vi "Robot Main.vi"() -> ()   [LabVIEW 2016]
doc: "This VI implements the framework and scheduler for your robotics program. It should not be necessary to modify the framework. You are expected to add your code to the VIs called from Robot Main - the ones located in the Team Code folder within the project."
uses:
  <vilib>/Rock Robotics/WPI/Camera/WPI_CameraImageSize.ctl
  NavX/_TypeDefs/FRIC_navX_DeviceNumbersTypeDef.ctl
  NavX/_TypeDefs/Z900_navX_SerialStreamTypeDef.ctl
  NavX/_Processing Loop/FRIC_navX_Internal_SPI_ProcessingLoop.vi
  NavX/_Processing Loop/FRIC_navX_Internal_USB_ProcessingLoop.vi
  _Support Files/Robot Global Data.vi
panel:
  in  "Image Size":T1=enum."320x240"
  in  "Enable Vision":bool
  in  "Finish":bool
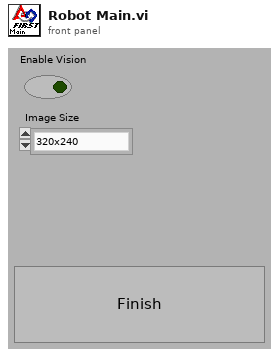
[diagram p1: front panel]
types:
  T1 = typedef "WPI_CameraImageSize.ctl" = enum16{"640x480", "320x240", "160x120", "Custom"}
  T2 = typedef "Z900_navX_SerialStreamTypeDef.ctl" = enum16{"YRPH", "Quaterinons", "Gyro/Raw", "AHRS", "AHRSAndPositioning"}
  T3 = typedef "FRIC_navX_DeviceNumbersTypeDef.ctl" = enum16{"Dev0", "Dev1", "Dev2", "Dev3", "Dev4", "Dev5", "Dev6", "Dev7", "Dev8", "Dev9", "Dev10"}
  T4 = typedef "WPI_DriverStationMatch Info.ctl" = cluster{"Autonomous Elapsed Seconds":dbl, "TeleOp Elapsed Seconds":dbl, "Disabled Elapsed Seconds":dbl, "Visited Autonomous":bool, "Visited TeleOp":bool, "Visited Disabled":bool, "Autonomous Settings":cluster{"Autonomous Style":enum16{"Iterative", "Independent"}, "VI Refnum":refnum<vi>}}
  T5 = typedef "WPI_DriverStationDerivedRobotMode.ctl" = enum16{"Init", "Execute", "Stop"}
  T6 = typedef "WPI_DriverStationRobotMode2.ctl" = enum16{"Autonomous Disabled", "Autonomous Enabled", "Teleop Disabled", "Teleop Enabled", "Disconnected", "Finish", "Test Disabled", "Test Enabled", "Emergency Stopped"}
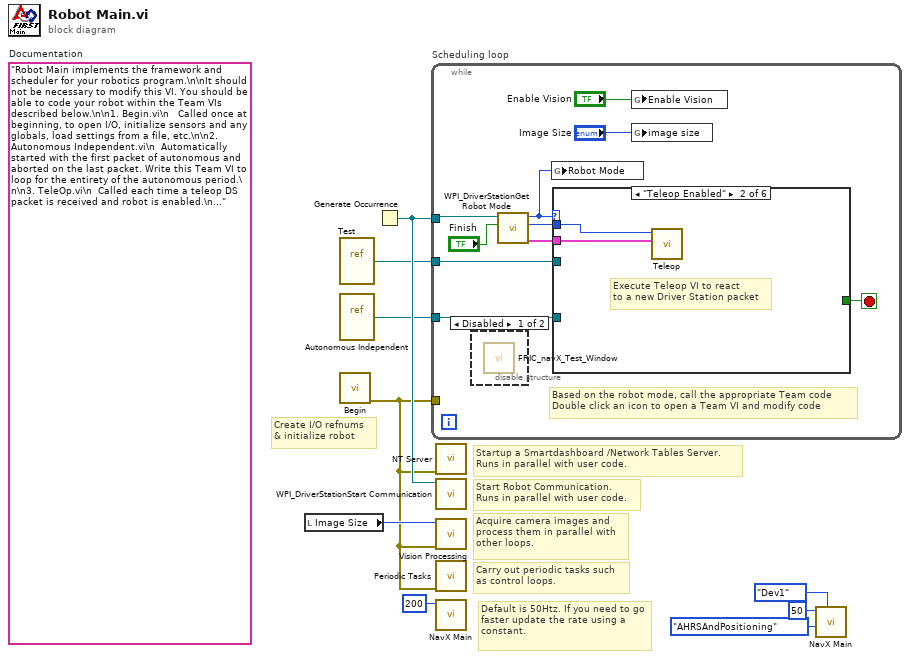
[diagram p0: block diagram]
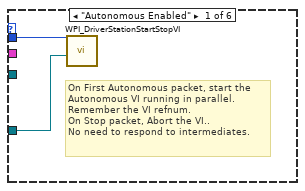
[diagram p3: hidden frame]
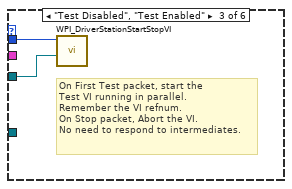
[diagram p4: hidden frame]
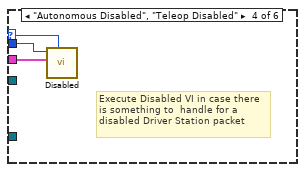
[diagram p5: hidden frame]
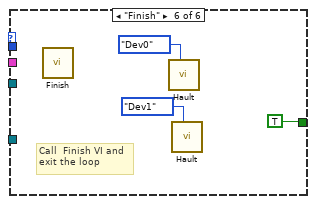
[diagram p7: hidden frame]
diagram:
  (unwired) "Robot Main implements the framework and scheduler for your robotics program.\n\nIt should not be necessary to modify this VI. You should be able to code your robot within the Team VIs described below.\n\n1. Begin.vi\n   Called once at beginning, to open I/O, initialize sensors and any globals, load settings from a file, etc.\n\n2. Autonomous Independent.vi\n  Automatically started with the first packet of autonomous and aborted on the last packet. Write this Team VI to loop for the entirety of the autonomous period.\n\n3. TeleOp.vi\n  Called each time a teleop DS packet is received and robot is enabled.\n\n4. Disabled.vi\n  Called each time a packet is received and the robot is disabled.\n\n5. Test.vi\n  Called Automatically started with the first test packet and aborted on the last. Modify this VI to carry out robot and sensor validation tests.\n\n6. Vision.vi\n  A parallel loop that acquires and processes camera images.\n\n7. PeriodicTasks.vi\n  Parallel loops running at user-defined rates.\n\n8. Finish.vi\n  Called before exiting, so you can save data, clean up I/O, etc.\n"  # Documentation
  # "Default is 50Htz. If you need to go faster update the rate using a constant."
  # "Startup a Smartdashboard /Network Tables Server.\nRuns in parallel with user code."
  # "Carry out periodic tasks such\nas control loops."
  # "Acquire camera images and\nprocess them in parallel with\nother loops."
  # "Create I/O refnums\n& initialize robot"
  # "Start Robot Communication.\nRuns in parallel with user code."
  n1 = local read "Image Size"() -> (w6:T1)
  n2 = vi-ref "Test.vi"() -> (w7:refnum<vi>)
  n3 = vi-ref "Autonomous Independent.vi"() -> (w8:refnum<vi>)
  n4 = call "Begin.vi"() -> ("error out"=w4:errorcluster)  [unwired: 1 in, 10 out]
  n5 = Generate Occurrence() -> (w9:refnum<k4>)
  n6 = while "Scheduling loop" {
    tunnel: w9 -> [w18]
    tunnel: w4 -> [_]
    tunnel: w8 -> [w13]
    tunnel: w7 -> [w11]
    stop <- w15 stop-if-true
    # "Based on the robot mode, call the appropriate Team code\nDouble click an icon to open a Team VI and modify code"
    n7 = disable-structure shown="Disabled" {
      frame Disabled {
        n8 = call "FRIC_navX_Test_Window.vi"() -> ()  [unwired: 12 in]
      }
      frame Enabled {
      }
    }
    n9 = call <vilib>:"WPI_DriverStationGet Robot Mode.vi"("Finish"="Finish", "DS Occurrence"=w18) -> ("Match Info out"=w16:T4, "Call Context"=w19:T5, "Robot Mode"=w10:T6)  [unwired: 7 out]
    n10 = global write "Robot Global Data.vi" "Robot Mode"(w10) -> ()
    n11 = case shown="\"Teleop Enabled\"" w10 {
      selector: w10 -> [_ _ _ w26 _ _]
      tunnel: w19 -> [w21 w23 w25 w28 _ _]
      tunnel: w16 -> [_ w22 _ w27 _ _]
      tunnel: [_ _ _ _ _ TRUE] -> w15
      tunnel: w13 -> [w20 _ _ _ _ _]
      tunnel: w11 -> [_ _ w24 _ _ _]
      frame "Autonomous Enabled" {
        # "On First Autonomous packet, start the\nAutonomous VI running in parallel.\nRemember the VI refnum.\nOn Stop packet, Abort the VI..\nNo need to respond to intermediates."
        n12 = call <vilib>:"WPI_DriverStationStartStopVI.vi"("VI in"=w20, "Call Context"=w21) -> ()  [unwired: 10 in]
      }
      frame "Teleop Enabled" {
        # "Execute Teleop VI to react\nto a new Driver Station packet"
        n13 = call "Teleop.vi"("Match Info"=w22, "Call Context"=w23) -> ()  [unwired: 1 in, 9 out]
      }
      frame "Test Disabled", "Test Enabled" {
        # "On First Test packet, start the\nTest VI running in parallel.\nRemember the VI refnum.\nOn Stop packet, Abort the VI.\nNo need to respond to intermediates."
        n14 = call <vilib>:"WPI_DriverStationStartStopVI.vi"("VI in"=w24, "Call Context"=w25) -> ()  [unwired: 10 in]
      }
      frame "Autonomous Disabled", "Teleop Disabled" {
        # "Execute Disabled VI in case there\nis something to  handle for a\ndisabled Driver Station packet"
        n15 = call "Disabled.vi"("Robot Mode"=w26, "Match Info"=w27, "Call Context"=w28) -> ()  [unwired: 1 in, 8 out]
      }
      frame "Disconnected", Default {
        # "Driver Station packet didn't arrive.\nPossibly useful for diagnostics"
      }
      frame "Finish" {
        # "Call  Finish VI and\nexit the loop"
        n16 = call "Finish.vi"() -> ()  [unwired: 1 in, 7 out]
        n17 = call "Hault.vi"("Device Number"=FRIC_navX_DeviceNumbersTypeDef."Dev0") -> ()  [unwired: 11 in]
        n18 = call "Hault.vi"("Device Number"=FRIC_navX_DeviceNumbersTypeDef."Dev1") -> ()  [unwired: 11 in]
      }
    }
    n19 = global write "Robot Global Data.vi" "Enable Vision"("Enable Vision") -> ()
    n20 = global write "Robot Global Data.vi" "image size"("Image Size") -> ()
  }
  n21 = call <vilib>:"NT Server.vi"("error in (no error)"=w4) -> ()  [unwired: 11 in]
  n22 = call <vilib>:"WPI_DriverStationStart Communication.vi"("occurrence"=w9) -> ()  [unwired: 1 in, 10 out]
  n23 = call "Vision Processing.vi"("error in (no error)"=w4, "Image Size"=w6) -> ()  [unwired: 6 out]
  n24 = call "Periodic Tasks.vi"("error in"=w4) -> ()  [unwired: 1 in, 10 out]
  n25 = call-poly "NavX Main.vi"("Rate (4Hz-200Hz)"=u8 200 ("Update Rate (4Hz-200Hz)")) -> ()  [unwired: 11 in]
  n26 = call-poly "NavX Main.vi"("Device Number"=FRIC_navX_DeviceNumbersTypeDef."Dev1", "Stream Type"=Z900_navX_SerialStreamTypeDef."AHRSAndPositioning", "Rate (4Hz-200Hz)"=u8 50) -> ()  [unwired: 9 in]
